vi "Measure Output.vi"(8 "error in":errorcluster, 11 "6032A in":refnum<class "6032A.lvclass">) -> (0 "error out":errorcluster, 1 "Current":dbl[](array[numeric]), 2 "Voltage":dbl[](array[numeric]), 3 "6032A out":refnum<class "6032A.lvclass">)   [LabVIEW 2019, in "6032A.lvlib" / "6032A.lvclass"]
doc: "Child classes must override this VI:\n\nThis VI is the device specific query of current and voltage measurements. \nThe return values are: \nVoltage Array - One voltage measurement per channel single channel supplies should only return a single array element\nCurrent Array - - One current measurement per channel single channel supplies should only return a single array element"
uses:
  Library/6032A.lvclass
  Library/6032A.lvclass/6032A.ctl
  <instrlib>/Agilent 6XXX Series/Agilent 6XXX Series.lvlib
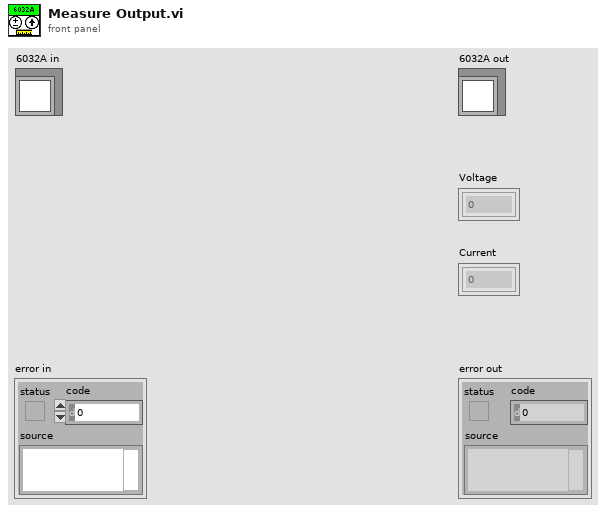
[diagram p1: front panel]
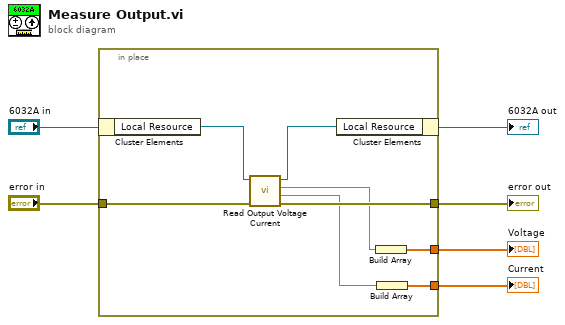
[diagram p0: block diagram]
diagram:
  n1 = in-place {
    in-place-border: "error in" -> [w12]
    in-place-border: [w11] -> w3
    in-place-border: [w8] -> w2
    in-place-border: [w7] -> w1
    n2 = in-place-cluster #1("6032A in") -> ("Local Resource"=w14:refnum<visa-resource-name>)
    n3 = call <instrlib>:"Read Output Voltage Current.vi"("error in (no error)"=w12, "VISA resource name"=w14) -> ("error out"=w11:errorcluster, "output current"=w9:dbl, "output voltage"=w10:dbl, "VISA resource name out"=w13:refnum<visa-resource-name>)  [unwired: 6 in]
    n4 = in-place-cluster #1("Local Resource"=w13) -> (→"6032A out":refnum<class "6032A.lvclass">)
    n5 = Build Array(w10) -> (w8:dbl[])
    n6 = Build Array(w9) -> (w7:dbl[])
  }
  "error out" <- w3
  "Current" <- w1
  "Voltage" <- w2
